vi "final_control_mk3_020825.vi"() -> ()   [LabVIEW 2023]
doc: "Simplified example program for initializing the COM port, determining the data frame of up to 26 Alicats, acquiring the data of the same number of Alicats, displaying the data of the one with the selected unit ID, and writing a setpoint to the same selected unit ID.\n\nThis is a slightly more feature rich version of the Alicat Simplified Driver Example, and contains an example of a method for interfacing with up to 26 Alicats on a single COM port by means of for loops with shift registers to handle sequential commands to each included Alicat. This also contains a method to write a setpoint to the same selected unit.\n\nIf coding for multiple Alicats on a single COM port without the use of for loops with shift registers, ensure that each Alicat command is executed sequentially. Alicat's RS-232/485 does not work if multiple devices are responding simultaneously."
uses:
  <vilib>/Platform/TimedLoop/XDataNode/timing_clust.ctl
  <vilib>/Platform/TimedLoop/XDataNode/nitl_modes.ctl
  <vilib>/Platform/TimedLoop/XDataNode/wakeup.ctl
  <vilib>/DAQmx/write.llb/DAQmx Write (Analog 1D DBL NChan 1Samp).vi
  <extravilib>/ChannelInstances/Tag-bool/Read With Abort.vi
  <extravilib>/ChannelInstances/Tag-bool/Write With Abort.vi
  <vilib>/Utility/file.llb/Write Delimited Spreadsheet (string).vi
  <extravilib>/ChannelInstances/Tag-bool/Instantiate.vi
  <extravilib>/ChannelInstances/Tag-bool/EndpointRead.vi
  <vilib>/DAQmx/miscellaneous.llb/DAQmx Fill In Error Info.vi
  <extravilib>/ChannelInstances/Tag-bool/Endpoint.vi
  <vilib>/platform/TimedLoop/XDataNode/XDataNode.xnode
  <vilib>/Platform/TimedLoop/XDataNode/XDNodeRunTimeDep.lvlib
  <extravilib>/ChannelInstances/Tag-bool.lvlib
panel:
  in  "End Program":bool
  in  "Tab Control":enum32{"Page 1", "Page 2"}(tab)
  in  "COM Port Settings":T1={"Baud Rate"=enum."19200", "VISA Sesssion In"="COM1"}
  out "Range Exceeded":bool
  out "Error Present":bool
  out "Error Text":string
  out "Elapsed Time [ms]\n(all units)":dbl caption="Elapsed Time (s)"
  in  "Minimum time between \nreadings [ms] (all units)":u32
  in  "Device ID's \nto Include:":T2={"A"=TRUE, "B"=FALSE, "C"=FALSE, "D"=FALSE, "E"=FALSE, "F"=FALSE, "G"=FALSE, "H"=FALSE, "I"=FALSE, "J"=FALSE, "K"=FALSE, "L"=FALSE, "M"=FALSE, "N"=FALSE, "O"=FALSE, "P"=FALSE, "Q"=FALSE, "R"=FALSE, "S"=FALSE, "T"=FALSE, "U"=FALSE, "V"=FALSE, "W"=FALSE, "X"=FALSE, "Y"=FALSE, "Z"=FALSE}
  out "Active Device":u16(ring) items=["A"]
  out "Meas. Data (for active device)":T3
  in  "file path":path=path "C:/Users/gtmiller/Downloads/Alicat LabVIEW 2014_2v1/Test.csv"
  out "len_SP":i32
  out "Setpoints":dbl[][](array[numeric])=[[4.2, 3.3], [69.0, 4.2]]
  out "N":i32
  out "Z":dbl[](array[numeric])
  # "Totalizer Timer"
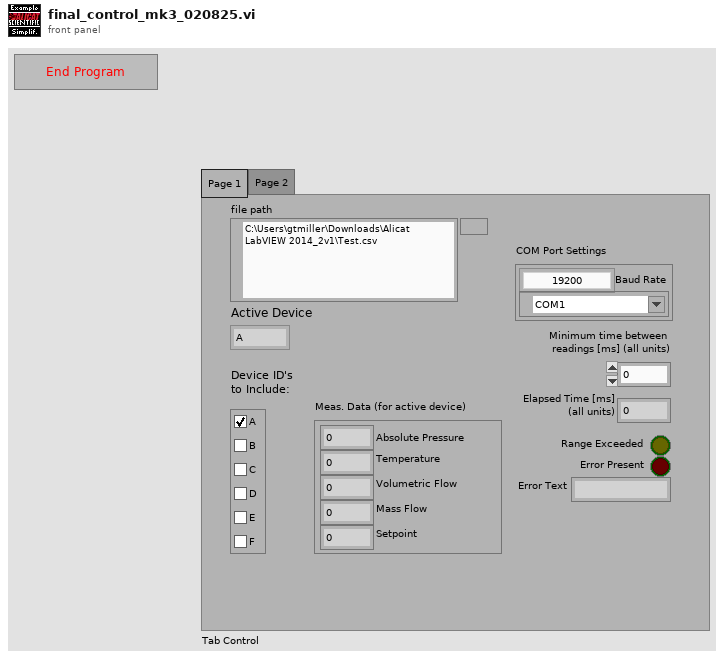
[diagram p1: front panel]
types:
  T1 = cluster{"Baud Rate":enum8{"2400", "9600", "19200", "38400", "57600", "115200", "Unknown"}, "VISA Sesssion In":refnum<visa-resource-name>}
  T2 = cluster{"A":bool, "B":bool, "C":bool, "D":bool, "E":bool, "F":bool, "G":bool, "H":bool, "I":bool, "J":bool, "K":bool, "L":bool, "M":bool, "N":bool, "O":bool, "P":bool, "Q":bool, "R":bool, "S":bool, "T":bool, "U":bool, "V":bool, "W":bool, "X":bool, "Y":bool, "Z":bool}
  T3 = cluster{"Absolute Pressure":dbl, "Gauge/Diff. Pressure":dbl, "Barometric Pressure":dbl, "Temperature":dbl, "Volumetric Flow":dbl, "Mass Flow":dbl, "Setpoint":dbl, "Valve Drive":dbl, "Totalizer":dbl, "[hr]":dbl, "[min]":dbl, "[sec]":dbl, "Totalizer Average Flow":dbl, "Totalizer Peak Flow":dbl, "Gas selected":string}
  T4 = cluster{"Unit ID":string, "Baud Rate":enum8{"2400", "9600", "19200", "38400", "57600", "115200", "Unknown"}, "VISA Sesssion In":refnum<visa-resource-name>}
  T5 = typedef "XDNodeRunTimeDep.lvlib/timing_clust.ctl" = cluster{"Expected End [f-1]":u64, "Actual End [f-1]":u64, "Finished Late? [f-1]":bool, "Expected End [i-1]":u64, "Actual End [i-1]":u64, "Finished Late? [i-1]":bool, "Expected Start [i]":u64, "Actual Start [i]":u64, "Expected Start [f]":u64, "Actual Start [f]":u64, "Source Name":string, "Structure Name":string, "Period":i64, "Deadline":i64, "Offset":i64, "Start":i64, "Priority":i32, "Timeout":i32, "Mode":T6, "Wakeup Reason":T7, "Error":errorcluster, "Source Type":string, "Secondary Source Type":string, "Global End Time":u64, "Global Start Time":u64, "Frame Duration":u64, "Iteration Duration":u64, "Assigned CPU":i32, "I/O Scan Engine Mode":u32}
  T6 = typedef "XDNodeRunTimeDep.lvlib/nitl_modes.ctl" = enum32{"No Change", "Process missed periods, maintain original phase", "Discard missed periods, maintain original phase", "Process missed periods, ignore original phase", "Discard missed periods, ignore original phase"}
  T7 = typedef "XDNodeRunTimeDep.lvlib/wakeup.ctl" = enum32{"Normal", "Aborted", "Asynchronous wakeup", "Timing source error", "Timed loop error", "Timeout"}
  T8 = enum8{"2400", "9600", "19200", "38400", "57600", "115200", "Unknown"}
  T9 = cluster{"Absolute Pressure":bool, "Gauge/Diff. Pressure":bool, "Barometric Pressure":bool, "Temperature":bool, "Volumetric":bool, "Mass":bool, "Setpoint":bool, "Valve Drive":bool, "Totalizer":bool, "Totalizer Timer":bool, "Totalizer Average Flow":bool, "Totalizer Peak Flow":bool, "Gas Selected":bool, "Tot. Timer Format":u16}
  T10 = cluster{"Controller Full Scale":dbl, "Controller Select":u16, "Control Range":enum16{"Normal", "Inverted", "Bidirectional", "Unknown"}}
  T11 = typedef "Tag-bool.lvlib/))Channel.ctl" = refnum<queue>
  T12 = cluster{"Controller Full Scale":dbl, "Controller Select":u16, "Control Range":enum16{"Normal", "Inverted", "Bidirectional", "Unknown"}}[]
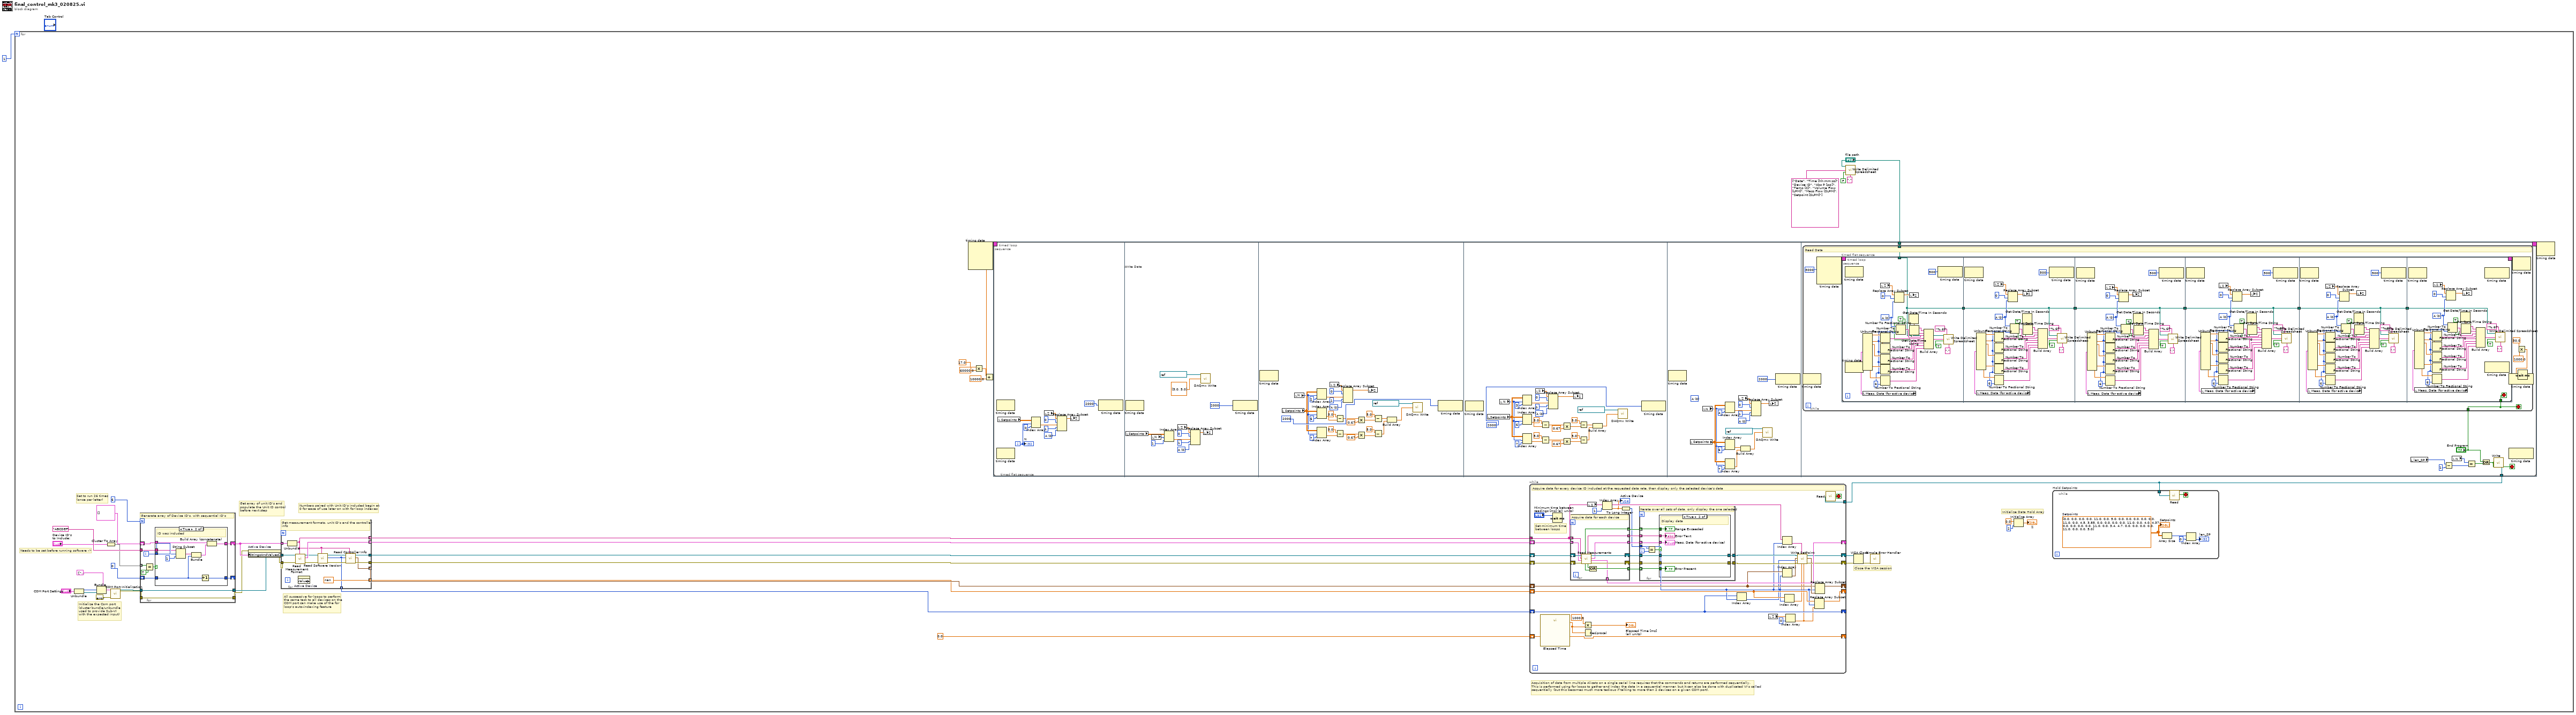
[diagram p0: block diagram]
diagram:
  n1 = for {
    N: 1 -> [_]
    # "Initialize Data Hold Array"
    # "All successive for loops to perform\nthe same task to all devices on the\nCOM port can make use of the for\nloop's auto-indexing feature"
    # "Set to run 26 times\n(once per letter)"
    # "Acquisition of data from multiple Alicats on a single serial line requires that the commands and returns are performed sequentially.\nThis is performed using for loops to gather and index the data in a sequential manner, but it can also be done with duplicated VI's called\nsequentially (but this becomes much more tedious if talking to more than 2 devices on a given COM port)."
    # "Numbers paired with Unit ID's included begin at\n0 for ease of use later on with for loop indexes"
    # "Get array of unit ID's and populate the Unit ID control before next step"
    # "Needs to be set before running software ->"
    # "Close the VISA session"
    # "Initialize the Com port\n(cluster bundle/unbundle\nused to provide Sub-VI \nwith the expected input)"
    n2 = Unbundle("COM Port Settings") -> ("Baud Rate"=w36:T8, "VISA Sesssion In"=w35:refnum<visa-resource-name>)
    n3 = Bundle(cluster=T4 {"Unit ID"="A", "Baud Rate"=enum."19200", "VISA Sesssion In"="COM1"} ("Communication Settings"), "Baud Rate"=w36, "VISA Sesssion In"=w35) -> (w34:T4)  [unwired: 1 in]
    n4 = Cluster To Array(cluster="Device ID's \nto Include:") -> (array=w30:bool[])
    n5 = call "COM Port Initialization.vi"("error in (no error)"=errorcluster {"status"=FALSE, "code"=0, "source"=""}, "Communication Settings"=w34) -> ("error out"=w27:errorcluster, "VISA Session Out"=w26:refnum<visa-resource-name>)  [unwired: 8 in]
    n6 = for {
      N: 6 -> [_]
      tunnel: "ABCDEF" -> [w418]
      tunnel: w30 -> [w411] mode=indexing
      shift-right: [w410] -> _
      shift-left: u16 0 ("length (rest)") -> [w416]
      shift-right: [w415] -> w24
      shift-left: cluster{string, u16}[] [] -> [w414]
      tunnel: w27 -> [w409]
      tunnel: w26 -> [w408]
      tunnel: [w409] -> w17
      tunnel: [w408] -> w25
      i -> [w417]
      # "Generate array of Device ID's, with sequential ID's"
      n7 = Equal?(x=w411, y=TRUE) -> (x = y?=w413:bool)
      n8 = case shown="True" w413 {
        tunnel: w418 -> [_ w429]
        tunnel: w417 -> [_ w428]
        tunnel: w416 -> [w419 w421]
        tunnel: [w420 w424] -> w415
        tunnel: w414 -> [w420 w422]
        tunnel: [w419 w425] -> w410
        frame False {
          # "ID was not included"
        }
        frame True {
          # "ID was included"
          n9 = String Subset(string=w429, offset (0)=w428, length (rest)=1 ("length (rest)")) -> (substring=w426:string)
          n10 = Bundle(w426, "length (rest)"=w421) -> (w423:cluster{string, "length (rest)":u16})  [unwired: 1 in]
          n11 = Increment(x=w421) -> (x+1=w425:u16)
          n12 = Build Array (concatenate)(w422, w423) -> (w424:cluster{string, "length (rest)":u16}[])
        }
      }
    }
    n13 = property on="Active Device" class="Ring (strict)"(error in=w17, "StringsAndValues[]"=w24) -> (error out=w16:errorcluster)  [unwired: 1 in, 1 out]
    n14 = for {
      tunnel: w25 -> [w406]
      tunnel: [w403] -> w21
      tunnel: w16 -> [w407]
      tunnel: [w402] -> w20
      tunnel: w24 -> [w404] mode=indexing
      tunnel: [w405] -> w23 mode=indexing
      tunnel: [w395] -> w22 mode=indexing
      tunnel: [w401] -> w19 mode=indexing
      tunnel: [nan ("Setpoint")] -> w18 mode=indexing
      tunnel: [w394] -> w15 mode=indexing
      # "Get measurement formats, unit ID's and the controller info"
      n15 = Unbundle(w404) -> (w395:string)  [unwired: 1 out]
      n16 = call "Read Measurement Format.vi"("Unit ID (A)"=w395, "error in"=w407, "VISA Session In"=w406) -> ("error out"=w398:errorcluster, "Data Frame Format"=w405:T9, "VISA Session Out"=w399:refnum<visa-resource-name>)  [unwired: 6 in]
      n17 = property on="Active Device" class="Ring (strict)" props=["Value"]() -> ()  [unwired: 2 in, 3 out]
      n18 = call "Read Software Version.vi"("Unit ID (A)"=w395, "error in"=w398, "VISA Session In"=w399) -> ("error out"=w397:errorcluster, "Software Version"=w394:u8, "VISA Session Out"=w396:refnum<visa-resource-name>)  [unwired: 6 in]
      n19 = call "Read Controller Info.vi"("Unit ID (A)"=w395, "error in"=w397, "Software Version"=w394, "VISA Session In"=w396) -> ("error out"=w402:errorcluster, "Controller Info out"=w401:T10, "VISA Session Out"=w403:refnum<visa-resource-name>)  [unwired: 4 in, 1 out]
    }
    n20 = Multiply(x=17.0, y=60000.0) -> (x*y=w8:dbl)
    n21 = Add(x=w8, y=10000.0) -> (x+y=w9:dbl)
    n22 = node-c288(w9) -> (w45:T5)  [unwired: 3 in]
    n23 = timed-loop "Write Data" {
      timing: w45 -> [_]
      timing-out: [_] -> w44
      tunnel: [w53] -> w11
      tunnel: "file path" -> [w52]
      i -> [w63]
      stop <- w174 stop-if-true
      n24 = timed-sequence {
        timing: _ -> [_]
        timing-out: _ -> [_]
        tunnel: [w55] -> w53
        tunnel: w52 -> [w54]
        n25 = timed-flat-sequence {
          tunnel: [w175] -> w55
          tunnel: w54 -> [w170]
          frame #0 {
            w56 = u16 0 items=["A", "B", "C", "D", "E", "F"]
            n26 = node-c288() -> ()  [unwired: 1 in, 1 out]
            n27 = local read "Setpoints"() -> (w65:dbl[][])
            n28 = Index Array(array=w65, index (row)=w63, index (col)=0 ("index (row)")) -> (element=w61:dbl)
            n29 = local read "Z"() -> (w59:dbl[])
            n30 = Replace Array Subset(array=w59, new element #1=w61, index #1=0 ("index"), new element #2=w56, index #2=1 ("index")) -> (w60:dbl[])
            n31 = local write "Z"(w60) -> ()
            n32 = node-c288(i64 2000 ("Start")) -> ()  [unwired: 1 out]
            "N" <- w63
          }
          frame #1 {
            w72 = u16 0 items=["A", "B", "C", "D", "E", "F"]
            n33 = node-c288() -> ()  [unwired: 1 in, 1 out]
            n34 = local read "Setpoints"() -> (w80:dbl[][])
            n35 = local read "N"() -> (w73:i32)
            n36 = Index Array(array=w80, index (row)=w73, index (col)=1 ("index (row)")) -> (element=w77:dbl)
            n37 = local read "Z"() -> (w75:dbl[])
            n38 = Replace Array Subset(array=w75, new element #1=w77, index #1=0 ("index"), new element #2=w72, index #2=1 ("index")) -> (w76:dbl[])
            n39 = call-poly <vilib>:"DAQmx Write.vi"("task/channels in"=refnum<k21> "Valve_cont", "data"=dbl[] [5.0, 5.0]) -> ()  [unwired: 11 in, 3 out]
            n40 = local write "Z"(w76) -> ()
            n41 = node-c288(i64 2000 ("Start")) -> ()  [unwired: 1 out]
          }
          frame #2 {
            w106 = u16 0 items=["A", "B", "C", "D", "E", "F"]
            n42 = node-c288() -> ()  [unwired: 1 in, 1 out]
            n43 = local read "Setpoints"() -> (w89:dbl[][])
            n44 = local read "N"() -> (w88:i32)
            n45 = Index Array(array=w89, index (row)=w88, index (col)=2 ("index (row)")) -> (element=w110:dbl)
            n46 = Index Array(array=w89, index (row)=w88, index (col)=6 ("disabled index (col)")) -> (element=w87:dbl)
            n47 = Index Array(array=w89, index (row)=w88, index (col)=7 ("disabled index (col)")) -> (element=w86:dbl)
            n48 = local read "Z"() -> (w108:dbl[])
            n49 = Subtract(x=5.0, y=w87) -> (x-y=w103:dbl)
            n50 = Subtract(x=5.0, y=w86) -> (x-y=w98:dbl)
            n51 = Replace Array Subset(array=w108, new element #1=w110, index #1=0 ("index"), new element #2=w106, index #2=1 ("index")) -> (w109:dbl[])
            n52 = Multiply(x=w103, y=0.67) -> (x*y=w101:dbl)
            n53 = Multiply(x=w98, y=0.67) -> (x*y=w96:dbl)
            n54 = local write "Z"(w109) -> ()
            n55 = Subtract(x=5.0, y=w101) -> (x-y=w91:dbl)
            n56 = Subtract(x=5.0, y=w96) -> (x-y=w92:dbl)
            n57 = Build Array(w91, w92) -> (w90:dbl[])
            n58 = call-poly <vilib>:"DAQmx Write.vi"("task/channels in"=refnum<k21> "Valve_cont", "data"=w90) -> ()  [unwired: 11 in, 3 out]
            n59 = node-c288(i64 2000 ("Start")) -> ()  [unwired: 1 out]
          }
          frame #3 {
            w138 = u16 0 items=["A", "B", "C", "D", "E", "F"]
            n60 = node-c288() -> ()  [unwired: 1 in, 1 out]
            n61 = local read "Setpoints"() -> (w121:dbl[][])
            n62 = local read "N"() -> (w120:i32)
            n63 = Index Array(array=w121, index (row)=w120, index (col)=3 ("index (row)")) -> (element=w142:dbl)
            n64 = Index Array(array=w121, index (row)=w120, index (col)=6 ("disabled index (col)")) -> (element=w119:dbl)
            n65 = Index Array(array=w121, index (row)=w120, index (col)=7 ("disabled index (col)")) -> (element=w118:dbl)
            n66 = local read "Z"() -> (w140:dbl[])
            n67 = Subtract(x=5.0, y=w119) -> (x-y=w135:dbl)
            n68 = Subtract(x=5.0, y=w118) -> (x-y=w130:dbl)
            n69 = Replace Array Subset(array=w140, new element #1=w142, index #1=0 ("index"), new element #2=w138, index #2=1 ("index")) -> (w141:dbl[])
            n70 = Multiply(x=w135, y=0.67) -> (x*y=w133:dbl)
            n71 = Multiply(x=w130, y=0.67) -> (x*y=w128:dbl)
            n72 = local write "Z"(w141) -> ()
            n73 = Subtract(x=5.0, y=w133) -> (x-y=w123:dbl)
            n74 = Subtract(x=5.0, y=w128) -> (x-y=w124:dbl)
            n75 = Build Array(w123, w124) -> (w122:dbl[])
            n76 = call-poly <vilib>:"DAQmx Write.vi"("task/channels in"=refnum<k21> "Valve_cont", "data"=w122) -> ()  [unwired: 11 in, 3 out]
            n77 = node-c288(i64 2000 ("Start")) -> ()  [unwired: 1 out]
          }
          frame #4 {
            (unwired) u16 0 items=["A", "B", "C", "D", "E", "F"]
            w159 = u16 0 items=["A", "B", "C", "D", "E", "F"]
            n78 = node-c288() -> ()  [unwired: 1 in, 1 out]
            n79 = local read "Setpoints"() -> (w153:dbl[][])
            n80 = local read "N"() -> (w152:i32)
            n81 = Index Array(array=w153, index (row)=w152, index (col)=4 ("index (row)")) -> (element=w163:dbl)
            n82 = Index Array(array=w153, index (row)=w152, index (col)=6 ("disabled index (col)")) -> (element=w155:dbl)
            n83 = Index Array(array=w153, index (row)=w152, index (col)=7 ("disabled index (col)")) -> (element=w154:dbl)
            n84 = local read "Z"() -> (w161:dbl[])
            n85 = Build Array(w155, w154) -> (w151:dbl[])
            n86 = Replace Array Subset(array=w161, new element #1=w163, index #1=0 ("index"), new element #2=w159, index #2=1 ("index")) -> (w162:dbl[])
            n87 = call-poly <vilib>:"DAQmx Write.vi"("task/channels in"=refnum<k21> "Valve_cont", "data"=w151) -> ()  [unwired: 11 in, 3 out]
            n88 = local write "Z"(w162) -> ()
            n89 = node-c288(i64 2000 ("Start")) -> ()  [unwired: 1 out]
          }
          frame #5 {
            n90 = node-c288() -> ()  [unwired: 1 in, 1 out]
            n91 = while {
              tunnel: "End Program" -> [w183]
              tunnel: w170 -> [w182]
              stop <- w183 stop-if-true
              # "Read Data"
              n92 = node-c288(i64 3000 ("Period")) -> (w186:T5)  [unwired: 3 in]
              n93 = timed-loop {
                timing: w186 -> [_]
                timing-out: [_] -> w185
                tunnel: w183 -> [w188]
                tunnel: w182 -> [w187]
                stop <- w352 stop-if-true
                n94 = timed-sequence {
                  timing: _ -> [_]
                  timing-out: _ -> [_]
                  tunnel: w188 -> [w195]
                  tunnel: w187 -> [w194]
                  n95 = timed-flat-sequence {
                    tunnel: w194 -> [w196]
                    tunnel: [w196] -> w193
                    tunnel: w193 -> [w227]
                    tunnel: [w227] -> w192
                    tunnel: w192 -> [w258]
                    tunnel: [w258] -> w191
                    tunnel: w191 -> [w289]
                    tunnel: [w289] -> w190
                    tunnel: w190 -> [w320]
                    tunnel: [w320] -> w189
                    tunnel: w195 -> [w352]
                    tunnel: w189 -> [w351]
                    frame #0 {
                      w200 = u16 0 items=["A", "B", "C", "D", "E", "F"]
                      w201 = i16 6 ("precision (6)")
                      n96 = node-c288() -> ()  [unwired: 1 in, 1 out]
                      n97 = local read "Meas. Data (for active device)"() -> (w208:T3)
                      n98 = Unbundle(w208) -> ("Absolute Pressure"=w221:dbl, "Temperature"=w217:dbl, "Volumetric Flow"=w207:dbl, "Mass Flow"=w218:dbl, "Setpoint"=w219:dbl)  [unwired: 10 out]
                      n99 = local read "Z"() -> (w204:dbl[])
                      n100 = Number To Fractional String(number=w221, precision (6)=w201) -> (F-format string=w216:string)  [unwired: 2 in]
                      n101 = Number To Fractional String(number=w217, precision (6)=w201) -> (F-format string=w215:string)  [unwired: 2 in]
                      n102 = Number To Fractional String(number=w207, precision (6)=w201) -> (F-format string=w214:string)  [unwired: 2 in]
                      n103 = Number To Fractional String(number=w218, precision (6)=w201) -> (F-format string=w213:string)  [unwired: 2 in]
                      n104 = Number To Fractional String(number=w219, precision (6)=w201) -> (F-format string=w212:string)  [unwired: 2 in]
                      n105 = Replace Array Subset(array=w204, new element=w200, index=0) -> (w202:dbl[])
                      n106 = Number To Fractional String(number=w200, precision (6)=w201) -> (F-format string=w220:string)  [unwired: 2 in]
                      n107 = Get Date/Time In Seconds() -> (seconds since 1Jan1904=w206:timestamp)
                      n108 = Get Date/Time String(seconds (now)=w206, want seconds? (F)=TRUE) -> (date string=w205:string, time string=w222:string)  [unwired: 1 in]
                      n109 = local write "Z"(w202) -> ()
                      n110 = Build Array(w205, w222, w220, w216, w215, w214, w213, w212) -> (w209:string[])
                      n111 = node-c288(i64 500 ("Start")) -> ()  [unwired: 1 out]
                      n112 = call-poly <vilib>:"Write Delimited Spreadsheet.vi"("file path (dialog if empty)"=w196, "format (%s)"="%.6f" ("format (%.3f)"), "1D data"=w209, "append to file? (new file:F)"=TRUE, "delimiter (\\t)"="," ("delimiter (\\t)")) -> ()  [unwired: 9 in, 2 out]
                    }
                    frame #1 {
                      w234 = u16 0 items=["A", "B", "C", "D", "E", "F"]
                      w235 = i16 6 ("precision (6)")
                      n113 = node-c288() -> ()  [unwired: 1 in, 1 out]
                      n114 = local read "Meas. Data (for active device)"() -> (w232:T3)
                      n115 = Unbundle(w232) -> ("Absolute Pressure"=w252:dbl, "Temperature"=w248:dbl, "Volumetric Flow"=w239:dbl, "Mass Flow"=w249:dbl, "Setpoint"=w250:dbl)  [unwired: 10 out]
                      n116 = local read "Z"() -> (w231:dbl[])
                      n117 = Number To Fractional String(number=w252, precision (6)=w235) -> (F-format string=w247:string)  [unwired: 2 in]
                      n118 = Number To Fractional String(number=w248, precision (6)=w235) -> (F-format string=w246:string)  [unwired: 2 in]
                      n119 = Number To Fractional String(number=w239, precision (6)=w235) -> (F-format string=w245:string)  [unwired: 2 in]
                      n120 = Number To Fractional String(number=w249, precision (6)=w235) -> (F-format string=w244:string)  [unwired: 2 in]
                      n121 = Number To Fractional String(number=w250, precision (6)=w235) -> (F-format string=w243:string)  [unwired: 2 in]
                      n122 = Replace Array Subset(array=w231, new element=w234, index=0) -> (w230:dbl[])
                      n123 = Number To Fractional String(number=w234, precision (6)=w235) -> (F-format string=w251:string)  [unwired: 2 in]
                      n124 = Get Date/Time In Seconds() -> (seconds since 1Jan1904=w238:timestamp)
                      n125 = Get Date/Time String(seconds (now)=w238, want seconds? (F)=TRUE) -> (date string=w237:string, time string=w253:string)  [unwired: 1 in]
                      n126 = local write "Z"(w230) -> ()
                      n127 = Build Array(w237, w253, w251, w247, w246, w245, w244, w243) -> (w240:string[])
                      n128 = node-c288(i64 500 ("Start")) -> ()  [unwired: 1 out]
                      n129 = call-poly <vilib>:"Write Delimited Spreadsheet.vi"("file path (dialog if empty)"=w227, "format (%s)"="%.6f" ("format (%.3f)"), "1D data"=w240, "append to file? (new file:F)"=TRUE, "delimiter (\\t)"="," ("delimiter (\\t)")) -> ()  [unwired: 9 in, 2 out]
                    }
                    frame #2 {
                      w265 = u16 0 items=["A", "B", "C", "D", "E", "F"]
                      w266 = i16 6 ("precision (6)")
                      n130 = node-c288() -> ()  [unwired: 1 in, 1 out]
                      n131 = local read "Meas. Data (for active device)"() -> (w261:T3)
                      n132 = Unbundle(w261) -> ("Absolute Pressure"=w283:dbl, "Temperature"=w279:dbl, "Volumetric Flow"=w270:dbl, "Mass Flow"=w280:dbl, "Setpoint"=w281:dbl)  [unwired: 10 out]
                      n133 = Number To Fractional String(number=w283, precision (6)=w266) -> (F-format string=w278:string)  [unwired: 2 in]
                      n134 = Number To Fractional String(number=w279, precision (6)=w266) -> (F-format string=w277:string)  [unwired: 2 in]
                      n135 = Number To Fractional String(number=w270, precision (6)=w266) -> (F-format string=w276:string)  [unwired: 2 in]
                      n136 = Number To Fractional String(number=w280, precision (6)=w266) -> (F-format string=w275:string)  [unwired: 2 in]
                      n137 = Number To Fractional String(number=w281, precision (6)=w266) -> (F-format string=w274:string)  [unwired: 2 in]
                      n138 = local read "Z"() -> (w263:dbl[])
                      n139 = Replace Array Subset(array=w263, new element=w265, index=0) -> (w262:dbl[])
                      n140 = Number To Fractional String(number=w265, precision (6)=w266) -> (F-format string=w282:string)  [unwired: 2 in]
                      n141 = local write "Z"(w262) -> ()
                      n142 = Get Date/Time In Seconds() -> (seconds since 1Jan1904=w269:timestamp)
                      n143 = Get Date/Time String(seconds (now)=w269, want seconds? (F)=TRUE) -> (date string=w268:string, time string=w284:string)  [unwired: 1 in]
                      n144 = Build Array(w268, w284, w282, w278, w277, w276, w275, w274) -> (w271:string[])
                      n145 = node-c288(i64 500 ("Start")) -> ()  [unwired: 1 out]
                      n146 = call-poly <vilib>:"Write Delimited Spreadsheet.vi"("file path (dialog if empty)"=w258, "format (%s)"="%.6f" ("format (%.3f)"), "1D data"=w271, "append to file? (new file:F)"=TRUE, "delimiter (\\t)"="," ("delimiter (\\t)")) -> ()  [unwired: 9 in, 2 out]
                    }
                    frame #3 {
                      w296 = u16 0 items=["A", "B", "C", "D", "E", "F"]
                      w297 = i16 6 ("precision (6)")
                      n147 = node-c288() -> ()  [unwired: 1 in, 1 out]
                      n148 = local read "Meas. Data (for active device)"() -> (w294:T3)
                      n149 = Unbundle(w294) -> ("Absolute Pressure"=w314:dbl, "Temperature"=w310:dbl, "Volumetric Flow"=w301:dbl, "Mass Flow"=w311:dbl, "Setpoint"=w312:dbl)  [unwired: 10 out]
                      n150 = Number To Fractional String(number=w314, precision (6)=w297) -> (F-format string=w309:string)  [unwired: 2 in]
                      n151 = Number To Fractional String(number=w310, precision (6)=w297) -> (F-format string=w308:string)  [unwired: 2 in]
                      n152 = Number To Fractional String(number=w301, precision (6)=w297) -> (F-format string=w307:string)  [unwired: 2 in]
                      n153 = Number To Fractional String(number=w311, precision (6)=w297) -> (F-format string=w306:string)  [unwired: 2 in]
                      n154 = Number To Fractional String(number=w312, precision (6)=w297) -> (F-format string=w305:string)  [unwired: 2 in]
                      n155 = local read "Z"() -> (w293:dbl[])
                      n156 = Replace Array Subset(array=w293, new element=w296, index=0) -> (w292:dbl[])
                      n157 = Number To Fractional String(number=w296, precision (6)=w297) -> (F-format string=w313:string)  [unwired: 2 in]
                      n158 = Get Date/Time In Seconds() -> (seconds since 1Jan1904=w300:timestamp)
                      n159 = Get Date/Time String(seconds (now)=w300, want seconds? (F)=TRUE) -> (date string=w299:string, time string=w315:string)  [unwired: 1 in]
                      n160 = local write "Z"(w292) -> ()
                      n161 = Build Array(w299, w315, w313, w309, w308, w307, w306, w305) -> (w302:string[])
                      n162 = node-c288(i64 500 ("Start")) -> ()  [unwired: 1 out]
                      n163 = call-poly <vilib>:"Write Delimited Spreadsheet.vi"("file path (dialog if empty)"=w289, "format (%s)"="%.6f" ("format (%.3f)"), "1D data"=w302, "append to file? (new file:F)"=TRUE, "delimiter (\\t)"="," ("delimiter (\\t)")) -> ()  [unwired: 9 in, 2 out]
                    }
                    frame #4 {
                      w327 = u16 0 items=["A", "B", "C", "D", "E", "F"]
                      w328 = i16 6 ("precision (6)")
                      n164 = node-c288() -> ()  [unwired: 1 in, 1 out]
                      n165 = local read "Meas. Data (for active device)"() -> (w325:T3)
                      n166 = Unbundle(w325) -> ("Absolute Pressure"=w345:dbl, "Temperature"=w341:dbl, "Volumetric Flow"=w332:dbl, "Mass Flow"=w342:dbl, "Setpoint"=w343:dbl)  [unwired: 10 out]
                      n167 = local read "Z"() -> (w324:dbl[])
                      n168 = Number To Fractional String(number=w345, precision (6)=w328) -> (F-format string=w340:string)  [unwired: 2 in]
                      n169 = Number To Fractional String(number=w341, precision (6)=w328) -> (F-format string=w339:string)  [unwired: 2 in]
                      n170 = Number To Fractional String(number=w332, precision (6)=w328) -> (F-format string=w338:string)  [unwired: 2 in]
                      n171 = Number To Fractional String(number=w342, precision (6)=w328) -> (F-format string=w337:string)  [unwired: 2 in]
                      n172 = Number To Fractional String(number=w343, precision (6)=w328) -> (F-format string=w336:string)  [unwired: 2 in]
                      n173 = Replace Array Subset(array=w324, new element=w327, index=0) -> (w323:dbl[])
                      n174 = Number To Fractional String(number=w327, precision (6)=w328) -> (F-format string=w344:string)  [unwired: 2 in]
                      n175 = Get Date/Time In Seconds() -> (seconds since 1Jan1904=w331:timestamp)
                      n176 = Get Date/Time String(seconds (now)=w331, want seconds? (F)=TRUE) -> (date string=w330:string, time string=w346:string)  [unwired: 1 in]
                      n177 = local write "Z"(w323) -> ()
                      n178 = Build Array(w330, w346, w344, w340, w339, w338, w337, w336) -> (w333:string[])
                      n179 = node-c288(i64 500 ("Start")) -> ()  [unwired: 1 out]
                      n180 = call-poly <vilib>:"Write Delimited Spreadsheet.vi"("file path (dialog if empty)"=w320, "format (%s)"="%.6f" ("format (%.3f)"), "1D data"=w333, "append to file? (new file:F)"=TRUE, "delimiter (\\t)"="," ("delimiter (\\t)")) -> ()  [unwired: 9 in, 2 out]
                    }
                    frame #5 {
                      w358 = u16 0 items=["A", "B", "C", "D", "E", "F"]
                      w359 = i16 6 ("precision (6)")
                      n181 = node-c288() -> ()  [unwired: 1 in, 1 out]
                      n182 = local read "Meas. Data (for active device)"() -> (w356:T3)
                      n183 = Unbundle(w356) -> ("Absolute Pressure"=w376:dbl, "Temperature"=w372:dbl, "Volumetric Flow"=w363:dbl, "Mass Flow"=w373:dbl, "Setpoint"=w374:dbl)  [unwired: 10 out]
                      n184 = Number To Fractional String(number=w376, precision (6)=w359) -> (F-format string=w371:string)  [unwired: 2 in]
                      n185 = Number To Fractional String(number=w372, precision (6)=w359) -> (F-format string=w370:string)  [unwired: 2 in]
                      n186 = Number To Fractional String(number=w363, precision (6)=w359) -> (F-format string=w369:string)  [unwired: 2 in]
                      n187 = Number To Fractional String(number=w373, precision (6)=w359) -> (F-format string=w368:string)  [unwired: 2 in]
                      n188 = Number To Fractional String(number=w374, precision (6)=w359) -> (F-format string=w367:string)  [unwired: 2 in]
                      n189 = local read "Z"() -> (w355:dbl[])
                      n190 = Replace Array Subset(array=w355, new element=w358, index=0) -> (w354:dbl[])
                      n191 = Number To Fractional String(number=w358, precision (6)=w359) -> (F-format string=w375:string)  [unwired: 2 in]
                      n192 = Get Date/Time In Seconds() -> (seconds since 1Jan1904=w362:timestamp)
                      n193 = Get Date/Time String(seconds (now)=w362, want seconds? (F)=TRUE) -> (date string=w361:string, time string=w377:string)  [unwired: 1 in]
                      n194 = local write "Z"(w354) -> ()
                      n195 = Build Array(w361, w377, w375, w371, w370, w369, w368, w367) -> (w364:string[])
                      n196 = node-c288() -> ()  [unwired: 1 in, 1 out]
                      n197 = call-poly <vilib>:"Write Delimited Spreadsheet.vi"("file path (dialog if empty)"=w351, "format (%s)"="%.6f" ("format (%.3f)"), "1D data"=w364, "append to file? (new file:F)"=TRUE, "delimiter (\\t)"="," ("delimiter (\\t)")) -> ()  [unwired: 9 in, 2 out]
                    }
                  }
                }
                n198 = node-c288() -> ()  [unwired: 1 in, 1 out]
                n199 = node-c288() -> ()  [unwired: 1 in, 1 out]
              }
              n200 = node-c288(w185) -> ()  [unwired: 1 out]
              n201 = Multiply(x=30.0, y=1000.0) -> (x*y=w181:dbl)
              n202 = Wait (ms)(milliseconds to wait=w181) -> ()  [unwired: 1 out]
            }
            n203 = local read "len_SP"() -> (w173:i32)
            n204 = Subtract(x=w173, y=1) -> (x-y=w177:i32)
            n205 = local read "N"() -> (w172:i32)
            n206 = Equal?(x=w172, y=w177) -> (x = y?=w176:bool)
            n207 = Or(x="End Program", y=w176) -> (x .or. y?=w174:bool)
            n208 = call <extravilib>:"Write.vi"("element"=w174) -> ("channel"=w175:T11)  [unwired: 1 out]
            n209 = node-c288() -> ()  [unwired: 1 in, 1 out]
          }
        }
      }
      n210 = node-c288() -> ()  [unwired: 1 in, 1 out]
      n211 = node-c288() -> ()  [unwired: 1 in, 1 out]
    }
    n212 = while {
      shift-right: [w466] -> _
      shift-left: 0.0 ("Set Start Time (s)") -> [w469]
      shift-right: [w450] -> w39
      shift-left: w20 -> [w468]
      shift-right: [w451] -> w40
      shift-left: w21 -> [w467]
      tunnel: w22 -> [w443]
      shift-right: [w454] -> _
      shift-left: w23 -> [w461]
      shift-right: [w449] -> _
      shift-left: w19 -> [w447]
      shift-right: [w445] -> _
      shift-left: w18 -> [w444]
      shift-right: [w439] -> _
      shift-left: w15 -> [w439]
      tunnel: w11 -> [w437]
      stop <- w438 stop-if-true
      # "Set minimum time\nbetween loops"
      # "Acquire data for every device ID included at the requested data rate, then display only the selected device's data"
      n213 = call "Elapsed Time"("Set Start Time (s)"=w469) -> ("Get Start Time (s)"=w466:dbl, "Elapsed Time (s)"=w463:dbl)  [unwired: 11 in, 6 out]
      n214 = Wait (ms)(milliseconds to wait="Minimum time between \nreadings [ms] (all units)") -> ()  [unwired: 1 out]
      n215 = for {
        shift-right: [w498] -> w460
        shift-left: w468 -> [w501]
        shift-right: [w499] -> w459
        shift-left: w467 -> [w500]
        tunnel: w461 -> [w495] mode=indexing
        tunnel: w443 -> [w494] mode=indexing
        tunnel: [w493] -> w458 mode=indexing
        tunnel: [w492] -> w457 mode=indexing
        tunnel: [w491] -> w456 mode=indexing
        tunnel: [w490] -> w455 mode=indexing
        tunnel: [w489] -> w454 mode=indexing
        # "Acquire data for each device"
        n216 = call "Read Measurements.vi"("error in"=w501, "Data Frame Format In"=w495, "Unit ID (A)"=w494, "VISA Session In"=w500) -> ("error out"=w498:errorcluster, "Data Frame Format Out"=w489:T9, "Data Cluster"=w492:T3, "VISA Session Out"=w499:refnum<visa-resource-name>, "Unknown Dataframe Info"=w497:bool, "Error/Overrange/Unknown String"=w491:string, "Error Present"=w496:bool, "Range Exceeded"=w490:bool)
        n217 = Or(x=w497, y=w496) -> (x .or. y?=w493:bool)
      }
      n218 = Multiply(x=1000.0 ("y"), y=w463) -> (x*y=→"Elapsed Time [ms]\n(all units)":dbl)
      n219 = Reciprocal(x=w463) -> ()  [unwired: 1 out]
      n220 = local read "Z"() -> (w432:dbl[])
      n221 = Index Array(array=w432, index=1 ("index (row)")) -> (element=w430:dbl)
      "Active Device" <- w430
      n222 = To Long Integer(number=w430) -> (32bit integer=w441:i32)
      n223 = for {
        tunnel: w460 -> [w472]
        tunnel: [w471] -> w452
        tunnel: w459 -> [w473]
        tunnel: [w470] -> w453
        tunnel: w458 -> [w478] mode=indexing
        tunnel: w441 -> [w480]
        tunnel: w457 -> [w477] mode=indexing
        tunnel: w456 -> [w476] mode=indexing
        tunnel: w455 -> [w475] mode=indexing
        i -> [w479]
        # "Iterate over all sets of data, only display the one selected"
        n224 = Equal?(x=w480, y=w479) -> (x = y?=w474:bool)
        n225 = case shown="True" w474 {
          tunnel: w478 -> [_ w488]
          tunnel: w477 -> [_ w483]
          tunnel: w476 -> [_ w487]
          tunnel: w475 -> [_ w486]
          tunnel: w473 -> [w482 w484]
          tunnel: w472 -> [w481 w485]
          tunnel: [w481 w485] -> w471
          tunnel: [w482 w484] -> w470
          frame False {
            # "Do nothing"
          }
          frame True {
            # "Display data"
            "Range Exceeded" <- w486
            "Error Present" <- w488
            "Error Text" <- w487
            "Meas. Data (for active device)" <- w483
          }
        }
      }
      n226 = Index Array(array=w439, index=w441) -> (element=w440:u8)
      n227 = local read "Z"() -> (w436:dbl[])
      n228 = Index Array(array=w443, index=w441) -> (element=w442:string)
      n229 = Index Array(array=w447, index=w441) -> (element=w446:T10)
      n230 = Index Array(array=w444, index=w441) -> (element=w433:dbl)
      n231 = Index Array(array=w436, index=0) -> (element=w434:dbl)
      n232 = call "Write SetPoint.vi"("Setpoint"=w434, "Previous Setpoint"=w433, "Unit ID (A)"=w442, "error in"=w452, "Software Version"=w440, "Controller Info out"=w446, "VISA Session In"=w453) -> ("error out"=w450:errorcluster, "Controller Info out"=w448:T10, "VISA Session Out"=w451:refnum<visa-resource-name>)  [unwired: 1 in, 1 out]
      n233 = Replace Array Subset(array=w444, new element=w434, index=w441) -> (w445:dbl[])
      n234 = Replace Array Subset(array=w447, new element=w448, index=w441) -> (w449:T12)
      n235 = call <extravilib>:"Read.vi"("channel"=w437) -> ("element"=w438:bool)  [unwired: 1 in, 1 out]
    }
    n236 = call-poly <vilib>:"Write Delimited Spreadsheet.vi"("file path (dialog if empty)"="file path", "1D data"=string[] ["Date", "Time [hh:mm:ss]", "Device ID", "Abs P [psi]", "Temp [C]", "Volume Flow [LPM]", "Mass Flow [SLPM]", "Setpoint [SLPM]"], "append to file? (new file:F)"=FALSE, "delimiter (\\t)"="," ("delimiter (\\t)")) -> ()  [unwired: 10 in, 2 out]
    n237 = VISA Close(VISA resource name=w40, error in (no error)=w39) -> (error out=w41:errorcluster)
    n238 = call <vilib>:"Simple Error Handler.vi"("error in (no error)"=w41) -> ()  [unwired: 4 in, 5 out]
    n239 = Initialize Array(0.0 ("element"), 2 ("dimension size")) -> (→"Z":dbl[])
    n240 = while "Hold Setpoints" {
      tunnel: w11 -> [w46]
      stop <- w47 stop-if-true
      w51 = dbl[][] [[0.0, 0.0, 0.0, 0.0, 11.0, 0.0, 5.0, 0.0], [0.0, 0.0, 0.0, 0.0, 11.0, 0.0, 4.5, 3.85], [0.0, 0.0, 0.0, 0.0, 11.0, 0.0, 4.0, 4.37], [0.0, 0.0, 0.0, 0.0, 11.0, 0.0, 3.4, 4.7], [0.0, 0.0, 0.0, 0.0, 11.0, 0.0, 0.0, 5.0]]  # Setpoints
      n241 = Array Size(array=w51) -> (size(s)=w49:i32[])
      n242 = call <extravilib>:"Read.vi"("channel"=w46) -> ("element"=w47:bool)  [unwired: 1 in, 1 out]
      n243 = Index Array(array=w49, index=0) -> (element=→"len_SP":i32)
      "Setpoints" <- w51
    }
    n244 = node-c288(w44) -> ()  [unwired: 1 out]
  }
